vi "Pointer MAIN producer consumer.vi"() -> ()   [LabVIEW 2014]
uses:
  Ctrls/Data cluster.ctl
  <vilib>/Utility/inputDevices.llb/closeKeyboard.vi
  support/User Event - Stop/User Event - Stop.lvlib
  support/Message Queue/Message Queue.lvlib
panel:
  out "COMP-S loopback disable request":bool
  out "COMP-S ON":bool
  out "Diodes \ncable OFF":bool
  out "Version":string
  out "CloudDet\n  Active":bool
  in  "Sound":bool
  in  "Help":bool
  in  "Clouds":bool
  in  "Auto Balance":bool
  out "Loopback\n   Active":bool
  out "Clouds\n detected":bool
  in  "Loopback":bool
  out "AutoBal \n Active":bool
  in  "Tab Control":T1(tab)
  in  "Auto diode":bool
  in  "Speed Control":u8(slide)=1 min=1 max=8 step=1 scale=1.0..8.0 scale format="%1d"
  in  "PA°":u16 max=359
  in  "UP":bool caption="Solar disk to UP\n side of the image"
  in  "RIGHT":bool caption="Solar disk to RIGHT\n side of the image"
  in  "DOWN":bool caption="Solar disk to DOWN\n side of the image"
  in  "LEFT":bool caption="Solar disk to LEFT\nside of the image"
  in  "CD_sensitivity %":i8(slide)=90 min=0 max=100 scale=0.1..100.0
  out "A+    Right diode":dbl format="%#.4g"
  out "D+    Bottom diode":dbl format="%#.4g"
  out "A-    Left diode":dbl format="%#.4g"
  out "D-     Upper diode":dbl caption="D-     Upper diode \nSouth@solar disk image" format="%#.4g"
  in  "Pointer \nTolerance":i8(slide)=1 min=1 max=100 step=1 scale=1.0..11.0
  in  "Diodes ON/OFF":bool=TRUE
  out "[V]":dbl=0.0023
  out "['']":i16
  in  "Default TDMS path":string="c:\\Pointer_logs_raw\\"
  in  "VISA port":refnum<visa-resource-name>="COM4"
  in  "PA Corr°":dbl caption="PA Correction°" min=-26.3 max=26.3 step=0.1 format="%#_3g"
  out "A+":bool
  out "A-":bool caption="A+"
  out "D+":bool caption="A+"
  out "D-":bool caption="A+"
  in  "Data Logging\n     ON/OFF":bool
  in  "Loops":u8=3 min=1
  out "TDMS file name/location":path
  out "Difference Chart":T2(graph)
  out "ADC Chart":cluster{dbl, dbl, dbl, dbl}(graph)
  out "Motor Chart":cluster{dbl, i16}(graph)
  out "Output picture":picture
  in  "Active num of impls":u8
  in  "Total num of impls":u8
  out "Impulses":bool
  out "Iteractions":i32
  out "HEX Out Cmd":string=" "
  out "PA rounded":dbl
  out "Speed level":u8
  in  "A+ ADC3":dbl=0.4 step=0.0025
  in  "D+ ADC2":dbl=0.4 step=0.0025
  in  "A-  ADC1":dbl=0.4 step=0.0025
  in  "D- ADC0":dbl=0.4 step=0.0025
  in  "Diodes - Manual":bool
  out "Vertical sum":dbl
  out "Horizontal sum":dbl
  in  "ADA  level 3 [V] in":dbl=0.2 format="%#_13g"
  in  "ADA  level 2 [V] in":dbl=0.05 format="%#_13g"
  out "ADA  level 1 [V]":dbl
  out "ADA  level 2 [V]":dbl
  in  "Reverse moving":bool=TRUE caption="Reverse \nmoving"
  out "ADA  level 3 [V]":dbl
  in  "ADA  level 1 [V] in":dbl=0.0023 format="%#_13g"
  out "max time":u32 caption="max process loop time [ms]"
  in  "Total stop":bool
  # "South@solar disk image"
  # "MOVING"
  # "East@solar disk image"
  # "West@solar disk image"
  # "North@solar disk image"
  # "View from the objective lens towards the primary solar image"
  # "MEASURED  VOLTAGES"
  # "MOTOR MOVING"
  # "SETTINGS"
  # "[%]"
  # "[~]"
  # "TDMS"
  # "For testing only"
  # "RM=False\nA0 -> STOP\nA1 -> DOWN\nA2 -> UP\nA4 -> RIGHT\nA8 -> LEFT\nA5 -> DOWN/RIGHT\nA6 -> UP/RIGHT\nA9 -> DOWN/LEFT\nAA -> UP/LEFT"
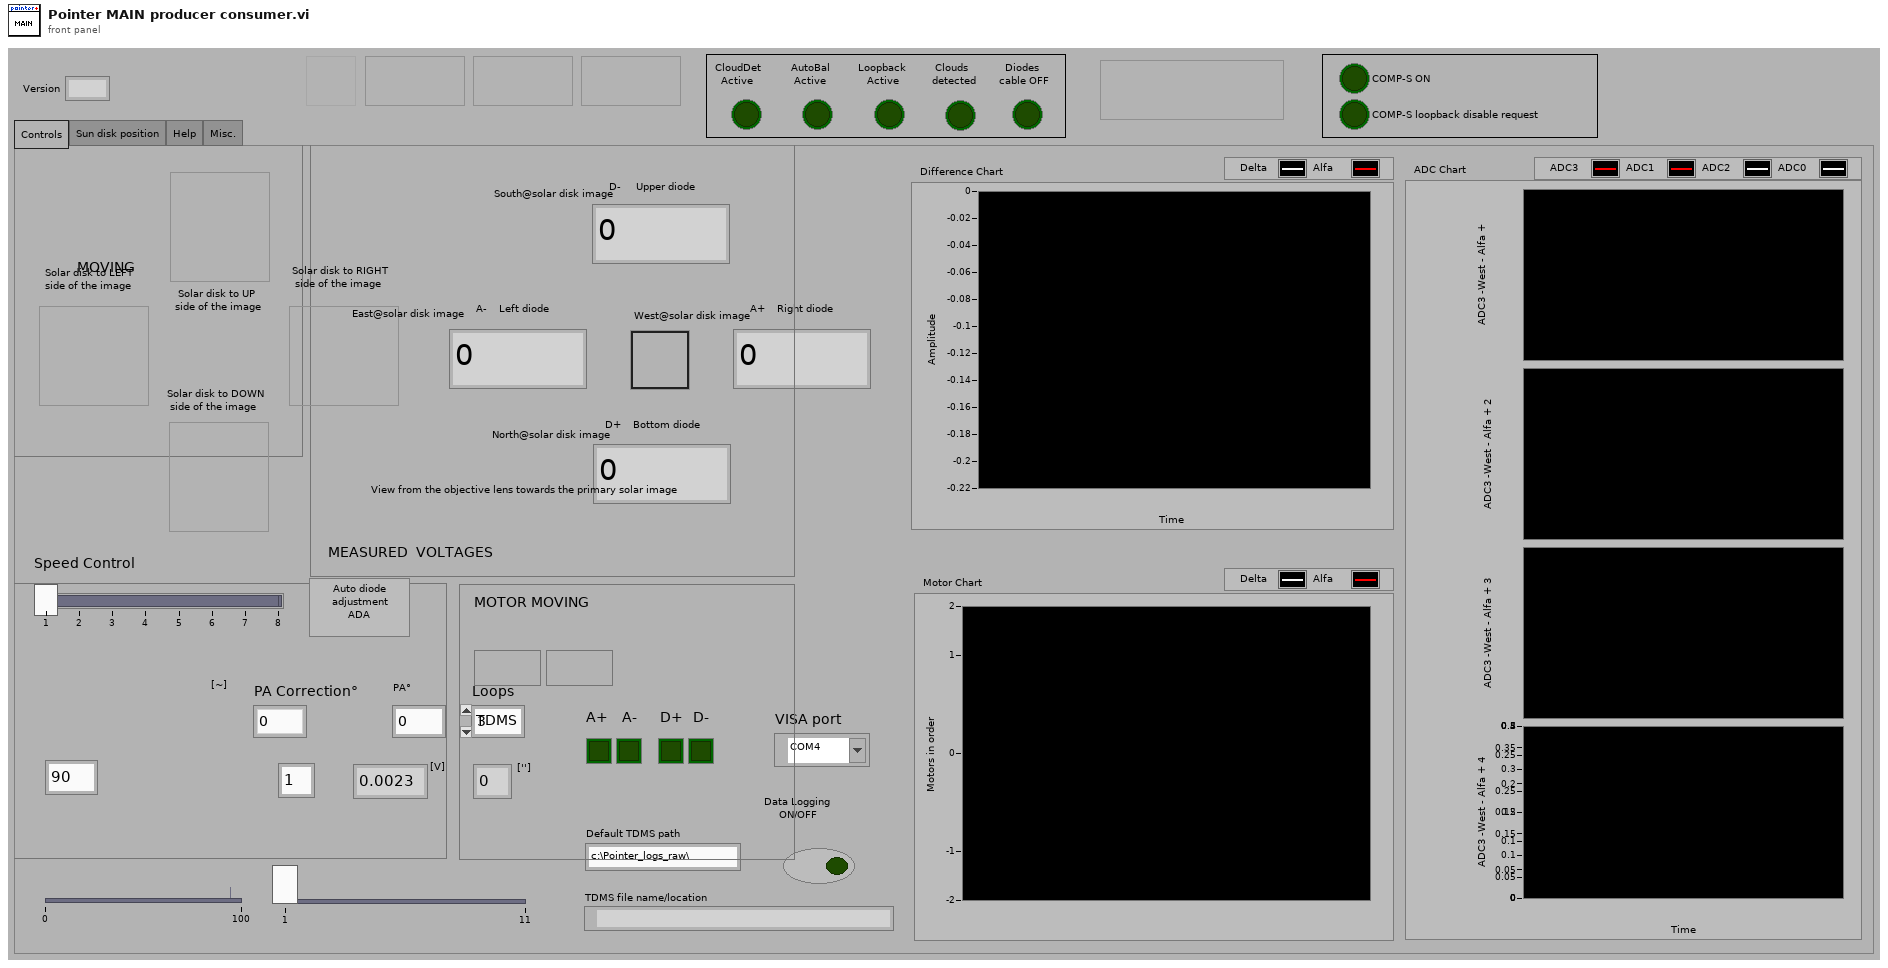
[diagram p1: front panel]
types:
  T1 = enum32{"Controls", "Sun disk position", "Help", "Misc."}
  T2 = cluster{"Vertical summary":dbl, "Horizontal summary":dbl}
  T3 = cluster{"Auto diode":refnum<vi>, "RIGHT":refnum<vi>, "UP":refnum<vi>, "LEFT":refnum<vi>, "DOWN":refnum<vi>, "Loopback":refnum<vi>, "Speed Control":refnum<vi>, "Data Log ON/OFF":refnum<vi>}
  T4 = typedef "Data cluster.ctl" = cluster{"[V]":dbl, "Vertical sum":dbl, "Horizontal sum":dbl, "auto Loopback":bool, "Auto Balance":bool, "Out Cmd":i32, "Motor Cmd":i32, "ADC Values":dbl[], "Clouds ctrl":bool, "Cloud Det":bool, "Cloud Sens":i8, "Loops":u8, "VISA res":refnum<visa-resource-name>}
  T5 = cluster{"Horizontal summary":dbl, "Vertical summary":dbl}[]
  T6 = cluster{"New ADC3":dbl, "New ADC2":dbl, dbl, dbl}[]
  T7 = typedef "LVDateTimeRec.ctl" = cluster{"fractional second":dbl, "second":i32, "minute":i32, "hour":i32, "day of month":i32, "month":i32, "year":i32, "day of week":i32, "day of year":i32, "DST":i32}
  T8 = typedef "Message Queue.lvlib/All Message Queues.ctl" = cluster{"UI":refnum<queue>}
  T9 = enum16{"0", "1", "2", "3", "4", "5", "6", "7", "8", "9", "A", "B", "C", "D", "E", "F", "G", "H", "I", "J", "K", "L", "M", "N", "O", "P", "Q", "R", "S", "T", "U", "V", "W", "X", "Y", "Z", "F1", "F2", "F3", "F4", "F5", "F6", "F7", "F8", "F9", "F10", "F11", "F12", "F13", "F14", "F15", "ADD", "BACK", "BACKSLASH", "CAPITAL", "COMMA", "DECIMAL", "DELETE", "DIVIDE", "DOWN", "END", "EQUALS", "ESCAPE", "GRAVE (`)", "HOME", "INSERT", "LBRACKET", "LCONTROL", "LEFT", "L ALT", "LSHIFT", "LWIN", "MINUS", "MULTIPLY", "NEXT", "NUMLOCK", "NUMPAD_0", "NUMPAD_1", "NUMPAD_2", "NUMPAD_3", "NUMPAD_4", "NUMPAD_5", "NUMPAD_6", "NUMPAD_7", "NUMPAD_8", "NUMPAD_9", "PAUSE", "PERIOD", "PRIOR (PG UP)", "RBRACKET", "RCONTROL", "RETURN", "RIGHT", "R ALT", "RSHIFT", "RWIN", "SCROLL", "SEMICOLON", "SLASH", "SPACE", "SUBTRACT", "TAB", "UP", "ENTER (num pad)", "' (quote)"}
  T10 = cluster{"Vertical sum":dbl, "Horizontal sum":dbl}
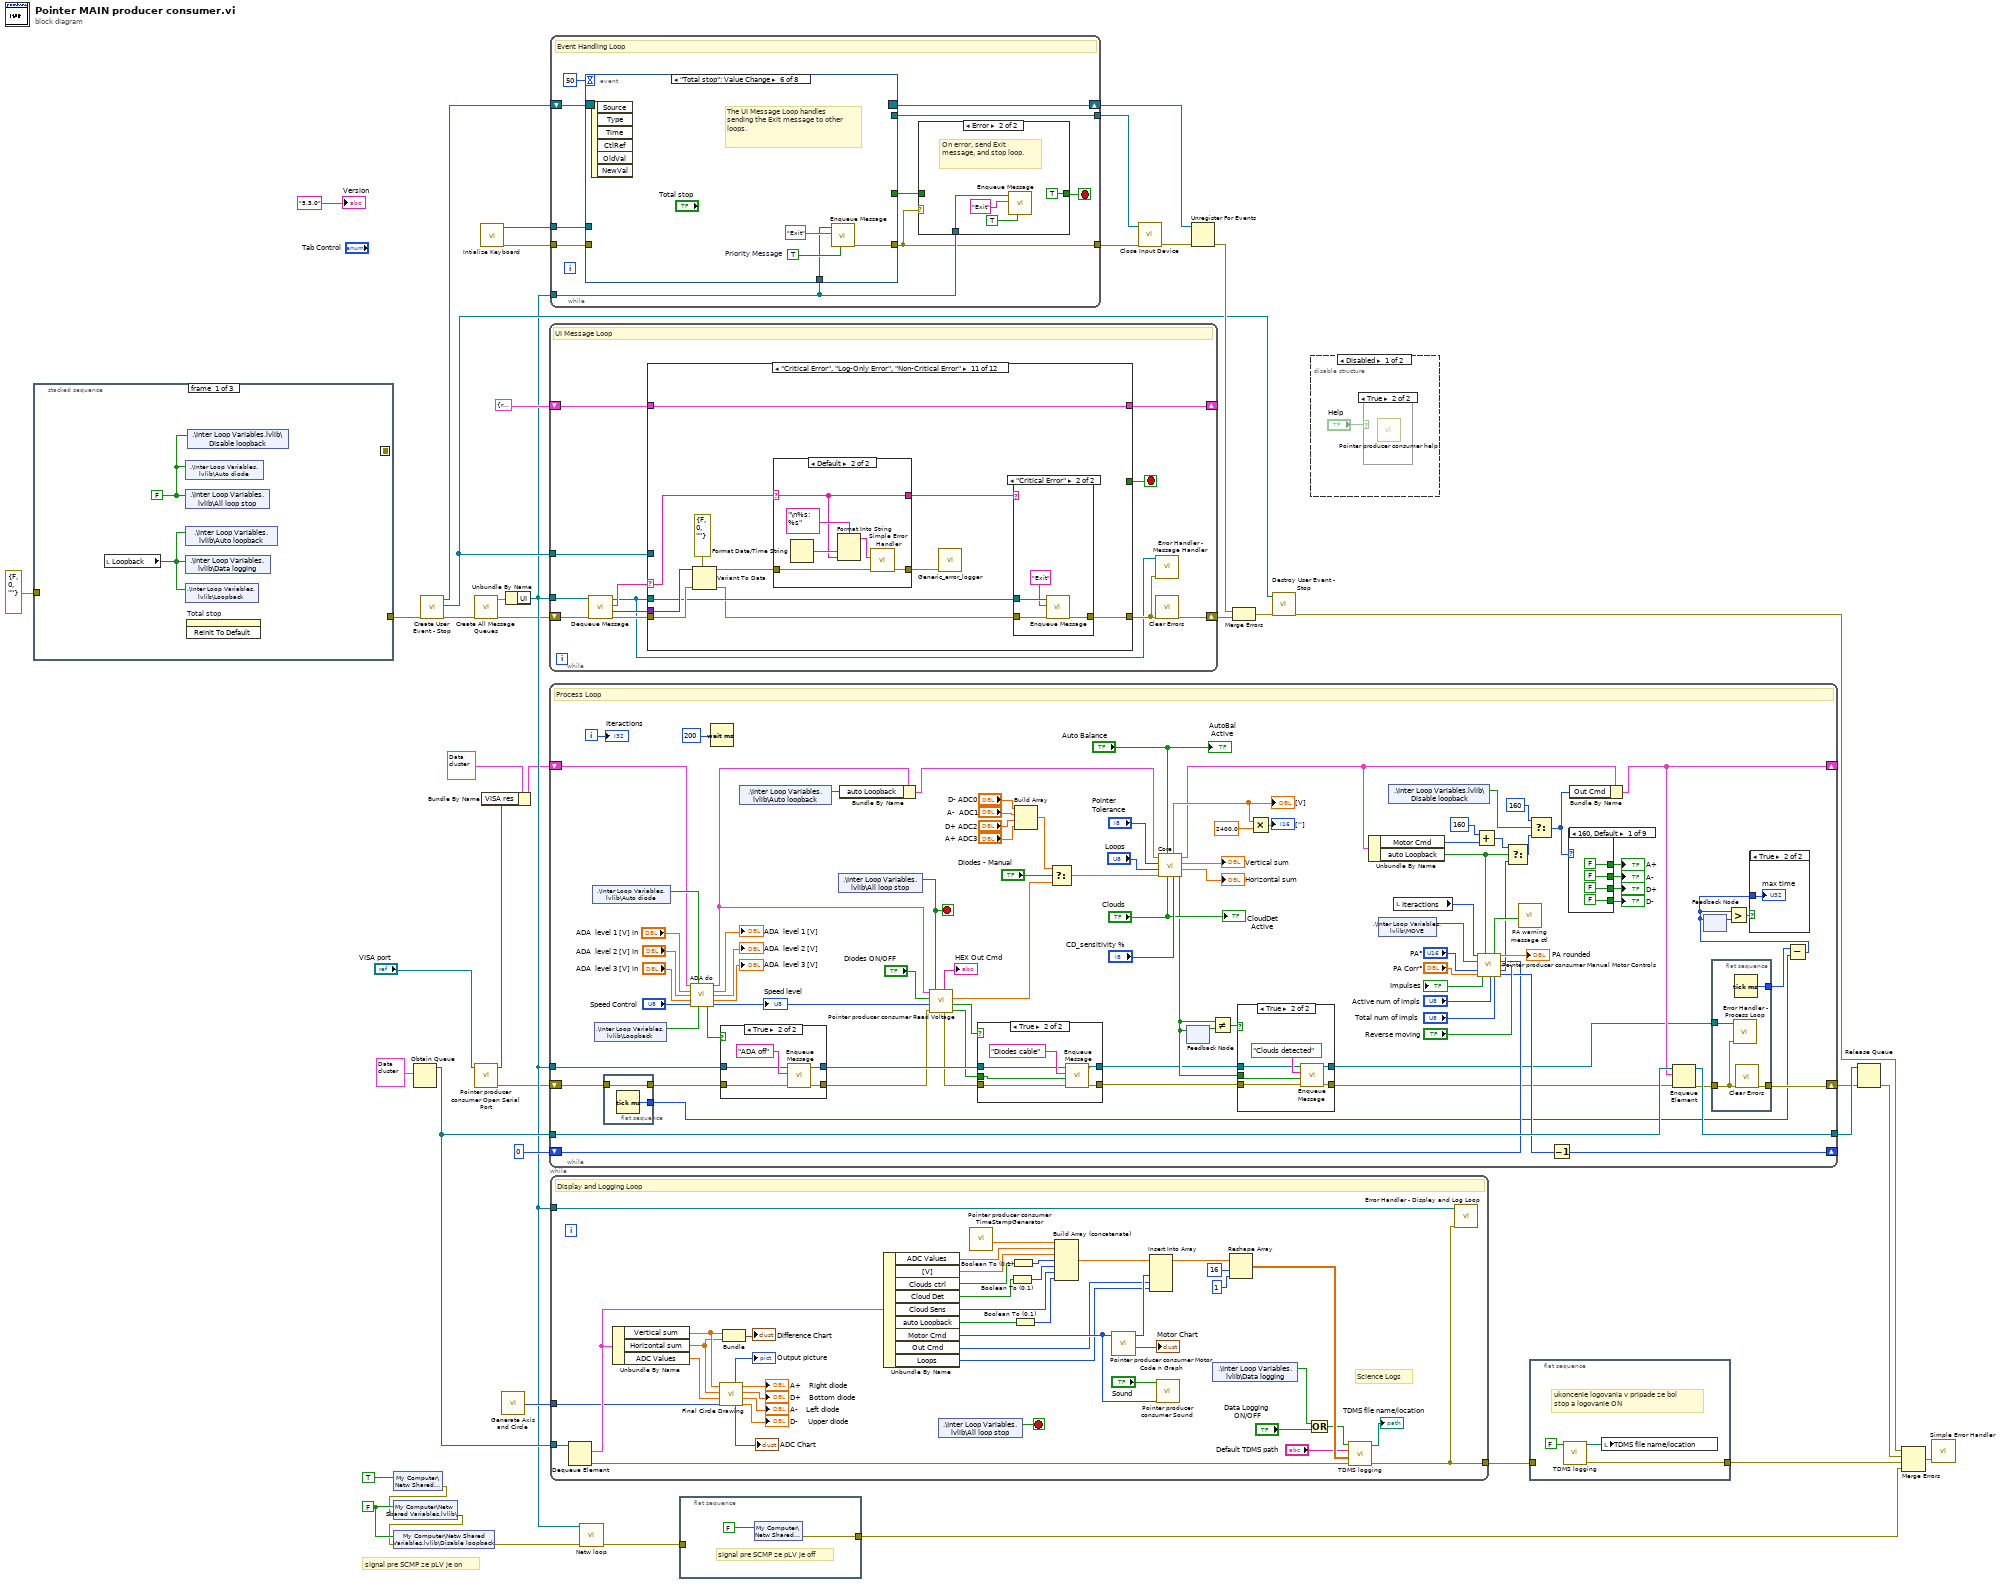
[diagram p0: block diagram]
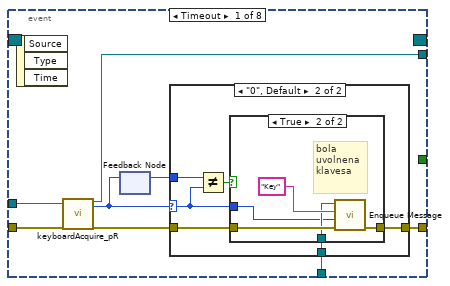
[diagram p5: hidden frame]
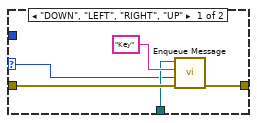
[diagram p6: hidden frame]
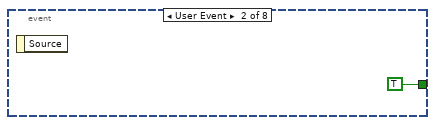
[diagram p8: hidden frame]
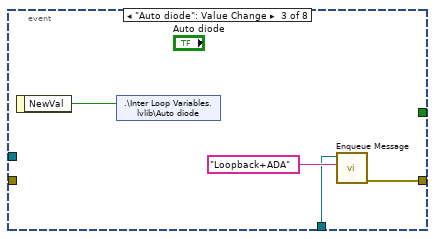
[diagram p9: hidden frame]
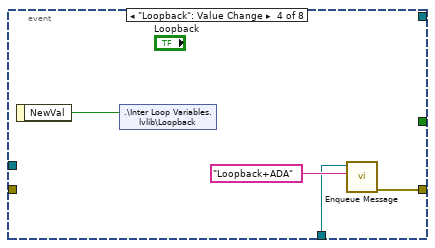
[diagram p10: hidden frame]
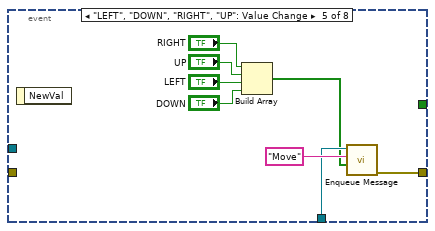
[diagram p11: hidden frame]
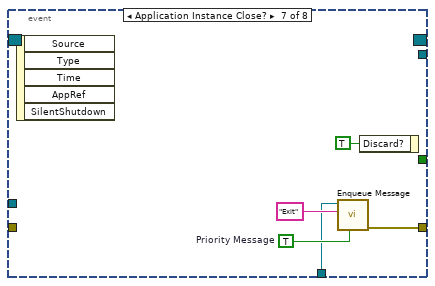
[diagram p12: hidden frame]
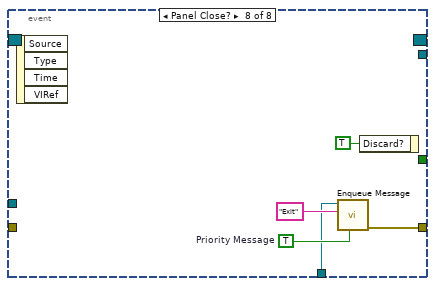
[diagram p13: hidden frame]
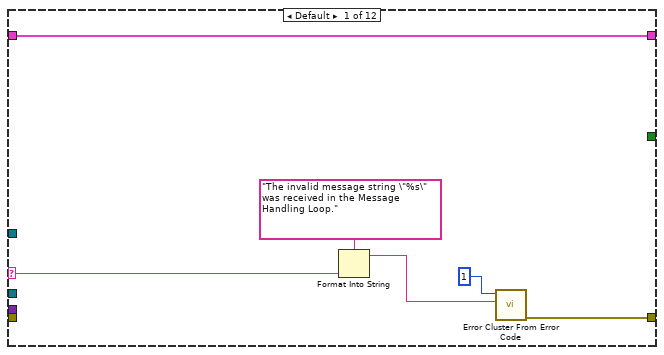
[diagram p14: hidden frame]
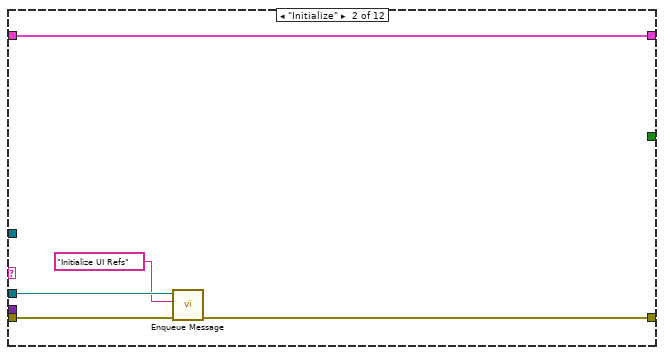
[diagram p15: hidden frame]
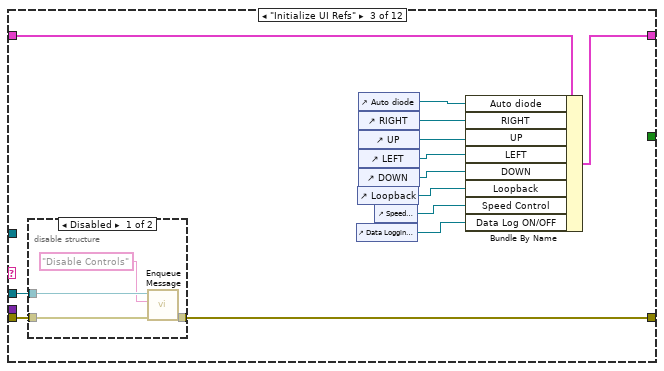
[diagram p16: hidden frame]
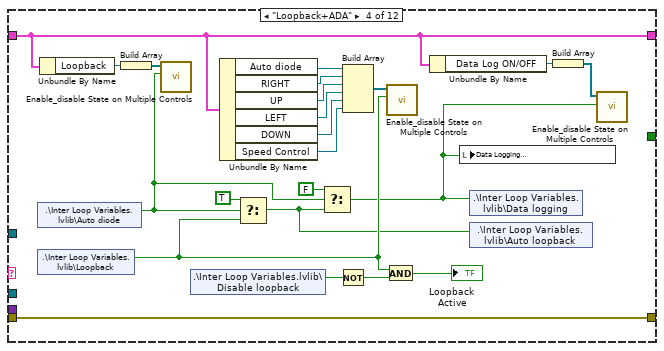
[diagram p18: hidden frame]
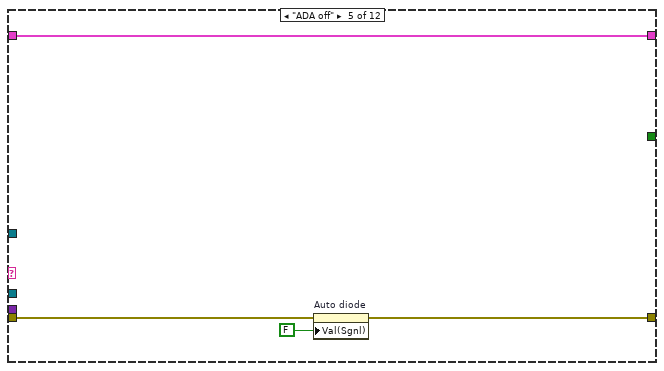
[diagram p19: hidden frame]
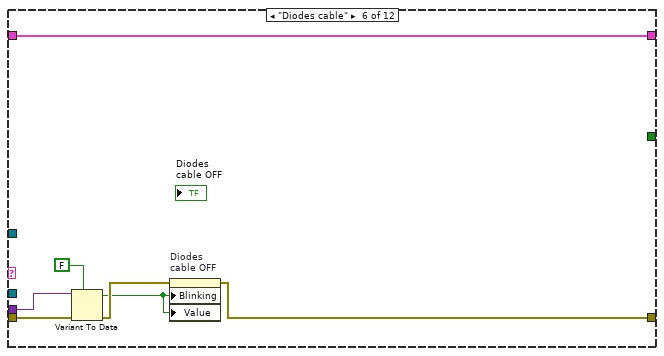
[diagram p20: hidden frame]
diagram:
  w11 = FALSE ("COMPs")
  # "signal pre SCMP ze pLV je on"
  n1 = stacked-sequence {
    seq-local: [_ w46 _] -> [_ _ w54]
    tunnel: [_ _ w57] -> w18
    tunnel: errorcluster {"status"=FALSE, "code"=0, "source"=""} ("error out") -> [_ w45 _]
    frame #0 {
      w43 = FALSE ("All loop stop")
      n2 = local read "Loopback"() -> (w44:bool)
      n3 = shared-variable ".\\Inter Loop Variables.lvlib\\Auto diode"(w43) -> ()  [unwired: 1 in, 1 out]
      n4 = shared-variable ".\\Inter Loop Variables.lvlib\\All loop stop"(w43) -> ()  [unwired: 1 in, 1 out]
      n5 = shared-variable ".\\Inter Loop Variables.lvlib\\Auto loopback"(w44) -> ()  [unwired: 1 in, 1 out]
      n6 = shared-variable ".\\Inter Loop Variables.lvlib\\Data logging"(w44) -> ()  [unwired: 1 in, 1 out]
      n7 = shared-variable ".\\Inter Loop Variables.lvlib\\Loopback"(w44) -> ()  [unwired: 1 in, 1 out]
      n8 = invoke on="Total stop" class="Bool" method="Reinit To Default"() -> ()  [unwired: 3 in, 3 out]
      n9 = shared-variable ".\\Inter Loop Variables.lvlib\\Disable loopback"(w43) -> ()  [unwired: 1 in, 1 out]
    }
    frame #1 {
      w49 = 0.200305 ("X Scale.Offset and Multiplier:Multiplier")
      # "mh v3.04: casova os -> akt cas"
      n10 = property on="Motor Chart" class="WFChart (strict)"(error in=w45, "XScale.Multiplier"=w49, "History Data"=cluster{i16, i16}[] [], "XScale.Maximum"=300.0 ("X Scale.Range:Maximum")) -> (error out=w48:errorcluster)  [unwired: 1 in, 1 out]
      n11 = property on="ADC Chart" class="WFChart (strict)"(error in=w48, "XScale.Multiplier"=w49, "History Data"=T6 []) -> (error out=w47:errorcluster)  [unwired: 1 in, 1 out]
      n12 = property on="Difference Chart" class="WFChart (strict)"(error in=w47, "XScale.Multiplier"=w49, "History Data"=T5 []) -> (error out=w46:errorcluster)  [unwired: 1 in, 1 out]
    }
    frame #2 {
      # "mh v3.04: casova os -> akt cas"
      n13 = Get Date/Time In Seconds() -> (seconds since 1Jan1904=w69:timestamp)
      n14 = Seconds To Date/Time(time stamp (now)=w69, to UTC (F)=TRUE) -> (date time rec=w68:T7)
      n15 = Unbundle(w68) -> ("second"=w62:i32, "minute"=w61:i32, "hour"=w60:i32)  [unwired: 7 out]
      n16 = Multiply(x=w60, y=60.0) -> (x*y=w67:dbl)
      n17 = Add(x=w61, y=w67) -> (x+y=w63:dbl)
      n18 = Multiply(x=w63, y=60.0) -> (x*y=w65:dbl)
      n19 = Add(x=w62, y=w65) -> (x+y=w58:dbl)
      n20 = property on="ADC Chart" class="WFChart (strict)"(error in=w54, "XScale.Offset"=w58) -> (error out=w55:errorcluster)  [unwired: 1 in, 1 out]
      n21 = property on="Difference Chart" class="WFChart (strict)"(error in=w55, "XScale.Offset"=w58) -> (error out=w56:errorcluster)  [unwired: 1 in, 1 out]
      n22 = property on="Motor Chart" class="WFChart (strict)"(error in=w56, "XScale.Offset"=w58) -> (error out=w57:errorcluster)  [unwired: 1 in, 1 out]
    }
  }
  n23 = shared-variable "My Computer\\Netw Shared Variables.lvlib\\pLV"(TRUE ("pLV")) -> (error out=w10:errorcluster)  [unwired: 1 in]
  n24 = shared-variable "My Computer\\Netw Shared Variables.lvlib\\COMPs"(w11, error in=w10) -> (error out=w9:errorcluster)
  n25 = shared-variable "My Computer\\Netw Shared Variables.lvlib\\Disable loopback"(w11, error in=w9) -> (error out=w8:errorcluster)
  n26 = Obtain Queue(element data type=T4 {"[V]"=0.0, "Vertical sum"=0.0, "Horizontal sum"=0.0, "auto Loopback"=FALSE, "Auto Balance"=FALSE, "Out Cmd"=0, "Motor Cmd"=0, "ADC Values"=[], "Clouds ctrl"=FALSE, "Cloud Det"=FALSE, "Cloud Sens"=0, "Loops"=0, "VISA res"="COM3"}) -> (queue out=w42:refnum<queue>)  [unwired: 4 in, 2 out]
  n27 = call "Create User Event - Stop.vi"("error in (no error)"=w18) -> ("error out"=w29:errorcluster, "User Event - Stop"=w24:refnum<user-event>, "Stop Event Registration Refnum"=w28:refnum<event-registration>)  [unwired: 8 in]
  n28 = call "Create All Message Queues.vi"("error in (no error)"=w29) -> ("error out"=w2:errorcluster, "Message Queues out"=w32:T8)  [unwired: 9 in]
  n29 = call "Pointer producer consumer Open Serial Port.vi"("VISA resource name"="VISA port") -> ("error out"=w1:errorcluster, "VISA resource name out"=w3:refnum<visa-resource-name>)  [unwired: 9 in]
  n30 = call <vilib>:"Intialize Keyboard.vi"() -> ("error out"=w21:errorcluster, "device ID"=w20:refnum<k1>)  [unwired: 1 in, 9 out]
  n31 = Bundle By Name(cluster=T4 {"[V]"=0.0, "Vertical sum"=0.0, "Horizontal sum"=0.0, "auto Loopback"=FALSE, "Auto Balance"=FALSE, "Out Cmd"=0, "Motor Cmd"=0, "ADC Values"=[], "Clouds ctrl"=FALSE, "Cloud Det"=FALSE, "Cloud Sens"=0, "Loops"=0, "VISA res"="COM3"}, "VISA res"=w3) -> (w4:T4)
  n32 = call "Generate Axis and Circle.vi"() -> ("Output picture"=w40:picture)  [unwired: 1 in]
  n33 = Unbundle By Name(w32) -> ("UI"=w13:refnum<queue>)
  n34 = while {
    shift-right: [w76] -> w31
    shift-left: w2 -> [w81]
    tunnel: w13 -> [w77]
    shift-right: [w72] -> _
    shift-left: T3 {"Auto diode"=refnum, "RIGHT"=refnum, "UP"=refnum, "LEFT"=refnum, "DOWN"=refnum, "Loopback"=refnum, "Speed Control"=refnum, "Data Log ON/OFF"=refnum} -> [w73]
    tunnel: w24 -> [w70]
    stop <- w71 stop-if-true
    # "UI Message Loop"
    n35 = call "Dequeue Message.vi"("error in (no error)"=w81, "Message Queue"=w77) -> ("error out"=w80:errorcluster, "Message Data"=w79:variant, "Message"=w78:string, "dup Message Queue"=w74:refnum<queue>)  [unwired: 6 in]
    n36 = case shown="\"Critical Error\", \"Log-Only Error\", \"Non-Critical Error\"" w78 {
      selector: w78 -> [w84 _ _ _ _ _ _ _ _ _ w200 _]
      tunnel: w80 -> [_ w91 w104 w130 w134 w142 w149 w158 w186 w197 w207 w230]
      tunnel: w79 -> [_ _ _ _ _ w141 w148 w157 w185 w196 w205 _]
      tunnel: w74 -> [_ w92 w105 _ _ _ _ w152 _ w188 w204 w225]
      tunnel: [w83 w90 w103 w130 w133 w137 w145 w153 w183 w189 w206 w228] -> w75
      tunnel: w73 -> [w82 w88 w94 w118 w136 w143 w150 w159 w187 w198 w209 w232]
      tunnel: [w82 w88 w93 w118 w136 w143 w150 w159 w187 w198 w209 w232] -> w72
      tunnel: [_ _ _ _ _ _ _ _ _ _ _ TRUE] -> w71
      tunnel: w70 -> [_ _ _ _ _ _ _ _ _ _ _ w227]
      frame Default {
        n37 = Format Into String(format string="The invalid message string \"%s\" was received in the Message Handling Loop." ("Invalid Message Loop Message"), w84) -> (resulting string=w85:string)  [unwired: 2 in, 1 out]
        n38 = call <vilib>:"Error Cluster From Error Code.vi"("error message (\"\")"=w85, "error code (0)"=1) -> ("error out"=w83:errorcluster)  [unwired: 7 in]
      }
      frame "Initialize" {
        n39 = call "Enqueue Message.vi"("error in (no error)"=w91, "Message"="Initialize UI Refs", "Message Queue"=w92) -> ("error out"=w90:errorcluster)  [unwired: 7 in, 1 out]
      }
      frame "Initialize UI Refs" {
        n40 = disable-structure shown="Disabled" {
          disable-tunnel: w105 -> [w109 _]
          disable-tunnel: w104 -> [w108 w110]
          disable-tunnel: [w107 w110] -> w103
          frame Disabled {
            n41 = call "Enqueue Message.vi"("error in (no error)"=w108, "Message"="Disable Controls", "Message Queue"=w109) -> ("error out"=w107:errorcluster)  [unwired: 7 in, 1 out]
          }
          frame Enabled {
          }
        }
        n42 = control-ref of="Data Logging ON/OFF"() -> (w102:refnum<vi>)
        n43 = control-ref of="Loopback"() -> (w100:refnum<vi>)
        n44 = control-ref of="Auto diode"() -> (w95:refnum<vi>)
        n45 = control-ref of="RIGHT"() -> (w96:refnum<vi>)
        n46 = control-ref of="UP"() -> (w97:refnum<vi>)
        n47 = control-ref of="LEFT"() -> (w98:refnum<vi>)
        n48 = control-ref of="DOWN"() -> (w99:refnum<vi>)
        n49 = control-ref of="Speed Control"() -> (w101:refnum<vi>)
        n50 = Bundle By Name(cluster=w94, "Auto diode"=w95, "RIGHT"=w96, "UP"=w97, "LEFT"=w98, "DOWN"=w99, "Loopback"=w100, "Speed Control"=w101, "Data Log ON/OFF"=w102) -> (w93:T3)
      }
      frame "Loopback+ADA" {
        n51 = shared-variable ".\\Inter Loop Variables.lvlib\\Auto diode"() -> (w127:bool)  [unwired: 1 in, 1 out]
        n52 = shared-variable ".\\Inter Loop Variables.lvlib\\Loopback"() -> (w119:bool)  [unwired: 1 in, 1 out]
        n53 = Unbundle By Name(w118) -> ("Loopback"=w132:refnum<vi>)
        n54 = Build Array(w132) -> (w131:refnum<vi>[])
        n55 = call "Enable_disable State on Multiple Controls.vi"("Disable control?"=w127, "Controls"=w131) -> ()  [unwired: 9 in, 1 out]
        n56 = shared-variable ".\\Inter Loop Variables.lvlib\\Disable loopback"() -> (w112:bool)  [unwired: 1 in, 1 out]
        n57 = Unbundle By Name(w118) -> ("Auto diode"=w121:refnum<vi>, "RIGHT"=w122:refnum<vi>, "UP"=w123:refnum<vi>, "LEFT"=w124:refnum<vi>, "DOWN"=w125:refnum<vi>, "Speed Control"=w126:refnum<vi>)
        n58 = Select(t=TRUE, s=w127, f=w119) -> (s? t:f=w115:bool)
        n59 = Select(t=FALSE, s=w127, f=w115) -> (s? t:f=w114:bool)
        n60 = Not(x=w112) -> (.not. x?=w111:bool)
        n61 = Build Array(w121, w122, w123, w124, w125, w126) -> (w120:refnum<vi>[])
        n62 = And(x=w119, y=w111) -> (x .and. y?=→"Loopback\n   Active":bool)
        n63 = call "Enable_disable State on Multiple Controls.vi"("Disable control?"=w119, "Controls"=w120) -> ()  [unwired: 9 in, 1 out]
        n64 = Unbundle By Name(w118) -> ("Data Log ON/OFF"=w116:refnum<vi>)
        n65 = local write "Data Logging\n     ON/OFF"(w114) -> ()
        n66 = shared-variable ".\\Inter Loop Variables.lvlib\\Data logging"(w114) -> ()  [unwired: 1 in, 1 out]
        n67 = shared-variable ".\\Inter Loop Variables.lvlib\\Auto loopback"(w115) -> ()  [unwired: 1 in, 1 out]
        n68 = Build Array(w116) -> (w117:refnum<vi>[])
        n69 = call "Enable_disable State on Multiple Controls.vi"("Disable control?"=w114, "Controls"=w117) -> ()  [unwired: 9 in, 1 out]
      }
      frame "ADA off" {
        n70 = property on="Auto diode" class="Bool (strict)"(error in=w134, "Val(Sgnl)"=FALSE) -> (error out=w133:errorcluster)  [unwired: 1 in, 1 out]
      }
      frame "Diodes cable" {
        n71 = Variant To Data(error in=w142, type=FALSE ("Diodes \ncable OFF"), Variant=w141) -> (data=w138:bool, error out=w139:errorcluster)
        n72 = property on="Diodes \ncable OFF" class="Bool (strict)"(error in=w139, "Blinking"=w138, "Value"=w138) -> (error out=w137:errorcluster)  [unwired: 1 in, 1 out]
      }
      frame "Clouds detected" {
        n73 = Variant To Data(error in=w149, type=FALSE ("Diodes \ncable OFF"), Variant=w148) -> (data=w144:bool, error out=w146:errorcluster)
        n74 = property on="Clouds\n detected" class="Bool (strict)"(error in=w146, "Blinking"=w144, "Value"=w144) -> (error out=w145:errorcluster)  [unwired: 1 in, 1 out]
      }
      frame "Key" {
        n75 = shared-variable ".\\Inter Loop Variables.lvlib\\Auto loopback"() -> (w151:bool)  [unwired: 1 in, 1 out]
        n76 = Variant To Data(error in=w158, type=T9."0" ("key pressed"), Variant=w157) -> (data=w155:T9, error out=w154:errorcluster)
        n77 = case shown="False" w151 {
          tunnel: w155 -> [w169 _]
          tunnel: w154 -> [w163 w181]
          tunnel: [w162 w181] -> w153
          tunnel: w152 -> [w161 _]
          frame False {
            n78 = case shown="\"0\", Default" w169 {
              tunnel: [w172 w174 w176 w178 w179] -> w165
              tunnel: [w172 w174 w176 w177 w180] -> w166
              tunnel: [w172 w173 w176 w178 w180] -> w168
              tunnel: [w172 w174 w175 w178 w180] -> w167
              tunnel: TRUE ("Solar disk to LEFT\nside of the image") -> [_ w173 w175 w177 w179]
              tunnel: FALSE ("Solar disk to LEFT\nside of the image") -> [w172 w174 w176 w178 w180]
              frame "0", Default {
                # "bola uvolnena klavesa"
              }
              frame "RIGHT" {
              }
              frame "UP" {
              }
              frame "LEFT" {
              }
              frame "DOWN" {
              }
            }
            n79 = local write "RIGHT"(w168) -> ()
            n80 = local write "UP"(w167) -> ()
            n81 = local write "LEFT"(w166) -> ()
            n82 = local write "DOWN"(w165) -> ()
            n83 = Build Array(w168, w167, w166, w165) -> (w160:bool[])
            n84 = call "Enqueue Message.vi"("error in (no error)"=w163, "Message Data"=w160, "Message"="Move", "Message Queue"=w161) -> ("error out"=w162:errorcluster)  [unwired: 6 in, 1 out]
          }
          frame True {
          }
        }
      }
      frame "Move" {
        n85 = Variant To Data(error in=w186, type=bool[] [TRUE, TRUE, TRUE, TRUE], Variant=w185) -> (data=w182:bool[], error out=w183:errorcluster)
        n86 = shared-variable ".\\Inter Loop Variables.lvlib\\MOVE"(w182) -> ()  [unwired: 1 in, 1 out]
      }
      frame "Netw Loopback" {
        # "volanie len kvoli update\n indikatoru loopback"
        n87 = Variant To Data(error in=w197, type=bool[] [TRUE, TRUE], Variant=w196) -> (data=w194:bool[], error out=w190:errorcluster)
        n88 = Index Array(array=w194) -> (element #1=→"COMP-S ON":bool, element #2=→"COMP-S loopback disable request":bool)  [unwired: 2 in]
        n89 = call "Enqueue Message.vi"("error in (no error)"=w190, "Message"="Loopback+ADA", "Message Queue"=w188) -> ("error out"=w189:errorcluster)  [unwired: 7 in, 1 out]
      }
      frame "Critical Error", "Log-Only Error", "Non-Critical Error" {
        n90 = Variant To Data(error in=w207, type=errorcluster {"status"=FALSE, "code"=0, "source"=""} ("error constant"), Variant=w205) -> (data=w202:errorcluster, error out=w203:errorcluster)
        n91 = case shown="Default" w200 {
          selector: w200 -> [w210 w212]
          tunnel: w202 -> [w211 w214]
          tunnel: [w211 w213] -> w201
          tunnel: [w210 w212] -> w199
          frame "Log-Only Error" {
          }
          frame Default {
            n92 = Format Date/Time String() -> (date/time string=w216:string)  [unwired: 3 in]
            n93 = Format Into String(format string="\n%s: %s", w216, w212) -> (resulting string=w215:string)  [unwired: 2 in, 1 out]
            n94 = call <vilib>:"Simple Error Handler.vi"("error source (\" \")"=w215, "error in (no error)"=w214) -> ("error out"=w213:errorcluster)  [unwired: 3 in, 4 out]
          }
        }
        n95 = call "Generic_error_logger.vi"("Error to log"=w201) -> ()  [unwired: 10 in, 1 out]
        n96 = case shown="\"Critical Error\"" w199 {
          tunnel: w203 -> [w218 w222]
          tunnel: w204 -> [_ w220]
          tunnel: [w218 w221] -> w206
          frame Default {
          }
          frame "Critical Error" {
            n97 = call "Enqueue Message.vi"("error in (no error)"=w222, "Message"="Exit", "Message Queue"=w220) -> ("error out"=w221:errorcluster)  [unwired: 7 in, 1 out]
          }
        }
      }
      frame "Exit" {
        w223 = FALSE ("COMP-S connected")
        # "Stop Event Handling Loop"
        # "Release the UI Message queue reference"
        # "Stop UI Message Loop"
        n98 = call "Fire User Event - Stop.vi"("User Event - Stop"=w227) -> ("error out"=w226:errorcluster)  [unwired: 10 in]
        n99 = Release Queue(queue=w225, error in (no error)=w230) -> (error out=w231:errorcluster)  [unwired: 1 in, 2 out]
        n100 = shared-variable ".\\Inter Loop Variables.lvlib\\All loop stop"(TRUE ("All loop stop")) -> ()  [unwired: 1 in, 1 out]
        n101 = local write "COMP-S loopback disable request"(w223) -> ()
        n102 = local write "COMP-S ON"(w223) -> ()
        n103 = Merge Errors(w226, w231) -> (w228:errorcluster)
      }
    }
    n104 = call "Error Handler - Message Handler.vi"("error in (no error)"=w75, "Message Queue"=w74) -> ()  [unwired: 9 in, 1 out]
    n105 = call <vilib>:"Clear Errors.vi"("error in (no error)"=w75) -> ("error out"=w76:errorcluster)  [unwired: 5 in, 1 out]
  }
  n106 = while {
    tunnel: w42 -> [w322]
    tunnel: [w321] -> w41
    shift-right: [w287] -> _
    shift-left: w4 -> [w246]
    shift-right: [w282] -> w37
    shift-left: w1 -> [w277]
    shift-right: [w290] -> _
    shift-left: 0 -> [w289]
    tunnel: w13 -> [w257]
    i -> [w320]
    stop <- w238 stop-if-true
    # "Process Loop"
    n107 = shared-variable ".\\Inter Loop Variables.lvlib\\Auto diode"() -> (w247:bool)  [unwired: 1 in, 1 out]
    n108 = shared-variable ".\\Inter Loop Variables.lvlib\\Loopback"() -> (w264:bool)  [unwired: 1 in, 1 out]
    n109 = flat-sequence {
      tunnel: [w332] -> w251
      tunnel: w277 -> [w332]
      tunnel: [w331] -> w250
      frame #0 {
        n110 = Tick Count (ms)() -> (millisecond timer value=w331:u32)
      }
    }
    n111 = call "ADA do.vi"("Data in"=w246, "Auto diode"=w247, "ADA  level 1 [V] in"="ADA  level 1 [V] in", "ADA  level 2 [V] in"="ADA  level 2 [V] in", "ADA  level 3 [V] in"="ADA  level 3 [V] in", "Speed Control in"="Speed Control", "Loopback"=w264) -> ("ADA off request"=w310:bool, "Data out"=w235:T4, "ADA  level 1 [V]"=→"ADA  level 1 [V]":dbl, "ADA  level 2 [V]"=→"ADA  level 2 [V]":dbl, "ADA  level 3 [V]"=→"ADA  level 3 [V]":dbl, "Speed Control out"=w233:u8)  [unwired: 3 in]
    "Speed level" <- w233
    n112 = Wait (ms)(milliseconds to wait=u32 200 ("Wait")) -> ()  [unwired: 1 out]
    n113 = case shown="True" w310 {
      tunnel: w257 -> [w383 w387]
      tunnel: [w383 w386] -> w256
      tunnel: [w382 w385] -> w237
      tunnel: w251 -> [w382 w384]
      frame False {
      }
      frame True {
        n114 = call "Enqueue Message.vi"("error in (no error)"=w384, "Message"="ADA off", "Message Queue"=w387) -> ("error out"=w385:errorcluster, "dup Message Queue"=w386:refnum<queue>)  [unwired: 7 in]
      }
    }
    n115 = shared-variable ".\\Inter Loop Variables.lvlib\\Auto loopback"() -> (w265:bool)  [unwired: 1 in, 1 out]
    n116 = shared-variable ".\\Inter Loop Variables.lvlib\\All loop stop"() -> (w238:bool)  [unwired: 1 in, 1 out]
    n117 = Bundle By Name(cluster=w235, "auto Loopback"=w265) -> (w245:T4)
    n118 = call "Pointer producer consumer Read Voltage.vi"("Total Stop"=w238, "error in (no error)"=w237, "Speed"=w233, "Diodes ON/OFF"="Diodes ON/OFF", "Data in"=w235) -> ("Diods cable OFF status"=w254:bool, "Diods cable OFF status request"=w255:bool, "ADC votlages"=w312:dbl[], "error out"=w236:errorcluster, "Motor Cmd"=→"HEX Out Cmd":string)  [unwired: 2 in]
    n119 = case shown="True" w255 {
      tunnel: w256 -> [w324 w329]
      tunnel: w236 -> [w323 w328]
      tunnel: w254 -> [_ w327]
      tunnel: [w324 w326] -> w253
      tunnel: [w323 w325] -> w252
      frame False {
      }
      frame True {
        n120 = call "Enqueue Message.vi"("error in (no error)"=w328, "Message Data"=w327, "Message"="Diodes cable", "Message Queue"=w329) -> ("error out"=w325:errorcluster, "dup Message Queue"=w326:refnum<queue>)  [unwired: 6 in]
      }
    }
    n121 = Build Array("D- ADC0", "A-  ADC1", "D+ ADC2", "A+ ADC3") -> (w314:dbl[])
    n122 = Select(t=w314, s="Diodes - Manual", f=w312) -> (s? t:f=w276:dbl[])
    n123 = call "Core.vi"("CD_sensitivity %"="CD_sensitivity %", "Clouds"="Clouds", "Auto Balance"="Auto Balance", "Real-time Values"=w276, "Loops"="Loops", "Pointer Tolerance"="Pointer \nTolerance", "Data in"=w245) -> ("Clouds detected"=w270:bool, "Horizontal sum"=→"Horizontal sum":dbl, "Vertical sum"=→"Vertical sum":dbl, "Data out"=w266:T4, "[V]"=w273:dbl)
    "[V]" <- w273
    n124 = feedback #1() -> (w285:bool)  [unwired: 1 in]
    n125 = feedback-in #1(w270) -> ()
    n126 = Not Equal?(x=w270, y=w285) -> (x != y?=w284:bool)
    n127 = case shown="True" w284 {
      tunnel: [w339 w341] -> w249
      tunnel: w270 -> [_ w342]
      tunnel: w253 -> [w338 w344]
      tunnel: w252 -> [w339 w343]
      tunnel: [w338 w340] -> w244
      frame False {
      }
      frame True {
        n128 = call "Enqueue Message.vi"("error in (no error)"=w343, "Message Data"=w342, "Message"="Clouds detected", "Message Queue"=w344) -> ("error out"=w341:errorcluster, "dup Message Queue"=w340:refnum<queue>)  [unwired: 6 in]
      }
    }
    n129 = Multiply(x=w273, y=2400.0) -> (x*y=→"['']":dbl)
    n130 = Unbundle By Name(w266) -> ("Motor Cmd"=w294:i32, "auto Loopback"=w288:bool)
    n131 = shared-variable ".\\Inter Loop Variables.lvlib\\MOVE"() -> (w248:bool[])  [unwired: 1 in, 1 out]
    n132 = shared-variable ".\\Inter Loop Variables.lvlib\\Disable loopback"() -> (w240:bool)  [unwired: 1 in, 1 out]
    n133 = local read "Iteractions"() -> (w301:i32)
    n134 = Add(x=160 ("y"), y=w294) -> (x+y=w299:i32)
    n135 = call "Pointer producer consumer Manual Motor Controls.vi"("Iteraction Counter"=w301, "loopback"=w288, "Input Array"=w248, "Impulse IN"=w289, "Reverse moving"="Reverse moving", "PA°"="PA°", "PA Correction°"="PA Corr°", "No. Impulses"="Active num of impls", "Modulo num"="Total num of impls") -> ("get info?"=w300:bool, "PA rounded"=→"PA rounded":dbl, "Output Number"=w292:i32, "Impulses"=→"Impulses":bool, "Impulse OUT"=w291:i32)  [unwired: 2 in]
    n136 = Select(t=w299, s=w288, f=w292) -> (s? t:f=w243:i32)
    n137 = call "PA warning message ctl.vi"("get info?"=w300) -> ()  [unwired: 11 in]
    n138 = Select(t=160 ("y"), s=w240, f=w243) -> (s? t:f=w242:i32)
    n139 = Decrement(x=w291) -> (x-1=w290:i32)
    n140 = case shown="160, Default" w242 {
      tunnel: [FALSE FALSE FALSE TRUE FALSE TRUE TRUE FALSE FALSE] -> w298
      tunnel: [FALSE FALSE FALSE FALSE TRUE FALSE FALSE TRUE TRUE] -> w297
      tunnel: [FALSE FALSE TRUE FALSE FALSE FALSE TRUE FALSE TRUE] -> w296
      tunnel: [FALSE TRUE FALSE FALSE FALSE TRUE FALSE TRUE FALSE] -> w295
      frame 160, Default {
      }
      frame 161 {
      }
      frame 162 {
      }
      frame 164 {
      }
      frame 168 {
      }
      frame 165 {
      }
      frame 166 {
      }
      frame 169 {
      }
      frame 170 {
      }
    }
    "A+" <- w298
    "A-" <- w297
    "D+" <- w296
    "D-" <- w295
    n141 = Bundle By Name(cluster=w266, "Out Cmd"=w242) -> (w287:T4)
    n142 = Enqueue Element(queue=w322, element=w287, error in (no error)=w249) -> (queue out=w321:refnum<queue>, error out=w283:errorcluster)  [unwired: 1 in, 1 out]
    n143 = feedback #2() -> (w280:u32)  [unwired: 1 in]
    n144 = flat-sequence {
      tunnel: [w336] -> w282
      tunnel: w283 -> [w335]
      tunnel: [w337] -> w281
      tunnel: w244 -> [w334]
      frame #0 {
        n145 = call "Error Handler - Process Loop.vi"("error in (no error)"=w335, "Message Queue"=w334) -> ()  [unwired: 9 in, 1 out]
        n146 = Tick Count (ms)() -> (millisecond timer value=w337:u32)
        n147 = call <vilib>:"Clear Errors.vi"("error in (no error)"=w335) -> ("error out"=w336:errorcluster)  [unwired: 5 in, 1 out]
      }
    }
    n148 = Subtract(x=w281, y=w250) -> (x-y=w279:u32)
    n149 = feedback-in #2(w279) -> ()
    n150 = Greater?(x=w279, y=w280) -> (0:w278:bool)
    n151 = case shown="True" w278 {
      tunnel: w279 -> [_ w333]
      frame False {
      }
      frame True {
        "max time" <- w333
      }
    }
    "Iteractions" <- w320
    "AutoBal \n Active" <- "Auto Balance"
    "CloudDet\n  Active" <- "Clouds"
  }
  n152 = while {
    shift-right: [w397] -> w27
    shift-left: w28 -> [w398]
    tunnel: w13 -> [w393]
    tunnel: w20 -> [w391]
    tunnel: [w390] -> w19
    tunnel: w21 -> [w392]
    tunnel: [w389] -> w17
    stop <- w396 stop-if-true
    # "Event Handling Loop"
    n153 = event shown="[5] \"Total stop\": Value Change" {
      selector: w398 -> [_ _ _ _ _ _ _ _]
      dyn-events: [_ _ _ _ _ _ _ _] -> w397
      timeout: 50 -> [_ _ _ _ _ _ _ _]
      tunnel: [_ TRUE ("Discard?") _ _ _ _ _ _] -> w395
      tunnel: [w408 _ w432 w436 w444 w447 w452 w457] -> w389
      tunnel: w393 -> [w406 _ w430 w434 w443 w446 w451 w456]
      tunnel: w392 -> [w411 _ _ _ _ _ _ _]
      tunnel: w391 -> [w410 _ _ _ _ _ _ _]
      tunnel: [w409 _ _ _ _ _ _ _] -> w390
      event Timeout {
        n154 = event-data() -> ()  [unwired: 1 in, 3 out]
        n155 = call "keyboardAcquire_pR.vi"("device ID"=w410, "error in (no error)"=w411) -> ("device ID"=w409:refnum<k1>, "key pressed"=w404:T9, "error out"=w407:errorcluster)  [unwired: 15 in]
        n156 = feedback-in #3(w404) -> ()
        n157 = feedback #3() -> (w405:T9)  [unwired: 1 in]
        n158 = case shown="\"0\", Default" w404 {
          selector: w404 -> [w412 w417]
          tunnel: [w415 w422] -> w408
          tunnel: w407 -> [w414 w421]
          tunnel: w406 -> [w413 w420]
          tunnel: w405 -> [_ w418]
          frame "DOWN", "LEFT", "RIGHT", "UP" {
            n159 = call "Enqueue Message.vi"("error in (no error)"=w414, "Message Data"=w412, "Message"="Key", "Message Queue"=w413) -> ("error out"=w415:errorcluster)  [unwired: 6 in, 1 out]
          }
          frame "0", Default {
            n160 = Not Equal?(x=w418, y=w417) -> (x != y?=w419:bool)
            n161 = case shown="True" w419 {
              tunnel: [w423 w427] -> w422
              tunnel: w421 -> [w423 w426]
              tunnel: w420 -> [_ w425]
              tunnel: w417 -> [_ w424]
              frame False {
              }
              frame True {
                # "bola uvolnena klavesa"
                n162 = call "Enqueue Message.vi"("error in (no error)"=w426, "Message Data"=w424, "Message"="Key", "Message Queue"=w425) -> ("error out"=w427:errorcluster)  [unwired: 6 in, 1 out]
              }
            }
          }
        }
      }
      event User Event {
        n163 = event-data() -> ()  [unwired: 1 in, 1 out]
      }
      event "Auto diode": Value Change {
        n164 = event-data() -> ("NewVal"=w431:bool)  [unwired: 1 in]
        n165 = shared-variable ".\\Inter Loop Variables.lvlib\\Auto diode"(w431) -> ()  [unwired: 1 in, 1 out]
        n166 = call "Enqueue Message.vi"("Message"="Loopback+ADA", "Message Queue"=w430) -> ("error out"=w432:errorcluster)  [unwired: 8 in, 1 out]
      }
      event "Loopback": Value Change {
        n167 = event-data() -> ("NewVal"=w435:bool)  [unwired: 1 in]
        n168 = shared-variable ".\\Inter Loop Variables.lvlib\\Loopback"(w435) -> ()  [unwired: 1 in, 1 out]
        n169 = call "Enqueue Message.vi"("Message"="Loopback+ADA", "Message Queue"=w434) -> ("error out"=w436:errorcluster)  [unwired: 8 in, 1 out]
      }
      event "LEFT", "DOWN", "RIGHT", "UP": Value Change {
        n170 = event-data() -> ()  [unwired: 1 in, 1 out]
        n171 = Build Array("RIGHT", "UP", "LEFT", "DOWN") -> (w438:bool[])
        n172 = call "Enqueue Message.vi"("Message Data"=w438, "Message"="Move", "Message Queue"=w443) -> ("error out"=w444:errorcluster)  [unwired: 7 in, 1 out]
      }
      event "Total stop": Value Change {
        w448 = TRUE  # Priority Message
        # "The UI Message Loop handles sending the Exit message to other loops."
        n173 = event-data() -> ()  [unwired: 1 in, 6 out]
        n174 = call "Enqueue Message.vi"("Priority Message? (F)"=w448, "Message"="Exit", "Message Queue"=w446) -> ("error out"=w447:errorcluster)  [unwired: 7 in, 1 out]
      }
      event Application Instance Close? {
        w453 = TRUE  # Priority Message
        n175 = event-data() -> ()  [unwired: 1 in, 5 out]
        n176 = call "Enqueue Message.vi"("Priority Message? (F)"=w453, "Message"="Exit", "Message Queue"=w451) -> ("error out"=w452:errorcluster)  [unwired: 7 in, 1 out]
        n177 = event-data("Discard?"=TRUE) -> ()  [unwired: 1 in, 1 out]
      }
      event Panel Close? {
        w458 = TRUE  # Priority Message
        n178 = event-data() -> ()  [unwired: 1 in, 4 out]
        n179 = call "Enqueue Message.vi"("Priority Message? (F)"=w458, "Message"="Exit", "Message Queue"=w456) -> ("error out"=w457:errorcluster)  [unwired: 7 in, 1 out]
        n180 = event-data("Discard?"=TRUE) -> ()  [unwired: 1 in, 1 out]
      }
    }
    n181 = case shown="Error" w389 {
      tunnel: [w399 TRUE ("Discard?")] -> w396
      tunnel: w395 -> [w399 _]
      tunnel: w393 -> [_ w400]
      frame No Error {
      }
      frame Error {
        # "On error, send Exit message, and stop loop."
        n182 = call "Enqueue Message.vi"("Priority Message? (F)"=TRUE ("Discard?"), "Message"="Exit", "Message Queue"=w400) -> ()  [unwired: 7 in, 2 out]
      }
    }
  }
  n183 = while {
    tunnel: w42 -> [w502]
    tunnel: w40 -> [w463]
    tunnel: w13 -> [w461]
    tunnel: [w460] -> w15
    stop <- w462 stop-if-true
    # "Science Logs"
    # "Display and Logging Loop"
    n184 = Dequeue Element(queue=w502) -> (element=w474:T4, error out=w465:errorcluster)  [unwired: 2 in, 2 out]
    n185 = Unbundle By Name(w474) -> ("Vertical sum"=w475:dbl, "Horizontal sum"=w472:dbl, "ADC Values"=w473:dbl[])
    n186 = call "Final Circle Drawing.vi"("picture"=w463, "Actual values"=w473, "Horizontal summary"=w472, "Vertical summary"=w475) -> ("ADC0"=→"D-     Upper diode":dbl, "ADC2"=→"A-    Left diode":dbl, "ADC1"=→"D+    Bottom diode":dbl, "ADC3"=→"A+    Right diode":dbl, "ADC Chart"=→"ADC Chart":cluster{dbl, dbl, dbl, dbl}, "Img result"=→"Output picture":picture)  [unwired: 2 in]
    n187 = Bundle("Vertical sum"=w475, "Horizontal sum"=w472) -> (→"Difference Chart":T10)  [unwired: 1 in]
    n188 = Unbundle By Name(w474) -> ("ADC Values"=w488:dbl[], "[V]"=w487:dbl, "Clouds ctrl"=w486:bool, "Cloud Det"=w484:bool, "Cloud Sens"=w482:i8, "auto Loopback"=w481:bool, "Motor Cmd"=w479:i32, "Out Cmd"=w478:i32, "Loops"=w477:u8)
    n189 = shared-variable ".\\Inter Loop Variables.lvlib\\All loop stop"() -> (w462:bool)  [unwired: 1 in, 1 out]
    n190 = call "Pointer producer consumer TimeStampGenerator.vi"() -> ("TIME Numeric"=w489:ext)  [unwired: 8 in, 2 out]
    n191 = Boolean To (0,1)(Boolean=w484) -> (0, 1=w483:i16)
    n192 = Boolean To (0,1)(Boolean=w486) -> (0, 1=w485:i16)
    n193 = Boolean To (0,1)(Boolean=w481) -> (0, 1=w480:i16)
    n194 = Build Array (concatenate)(w489, w488, w487, w485, w483, w482, w480) -> (w500:ext[])
    n195 = call "Pointer producer consumer Motor Code n Graph.vi"("DecimalMotorCode"=w479) -> ("Motor"=→"Motor Chart":cluster{dbl, i16}, "MotorSubarray"=w499:i16[])  [unwired: 6 in, 2 out]
    n196 = Insert Into Array(array=w500, new element #1=w499, new element #2=w478, new element #3=w477) -> (w476:ext[])  [unwired: 1 in]
    n197 = call "Pointer producer consumer Sound.vi"("Sound"="Sound", "Numeric"=w479) -> ()  [unwired: 9 in]
    n198 = shared-variable ".\\Inter Loop Variables.lvlib\\Data logging"() -> (w464:bool)  [unwired: 1 in, 1 out]
    n199 = Reshape Array(w476, 16 ("dimension size"), 1 ("dimension size")) -> (w493:ext[][])
    n200 = Or(x=w464, y="Data Logging\n     ON/OFF") -> (x .or. y?=w491:bool)
    n201 = call "TDMS logging.vi"("error in (no error)"=w465, "Data"=w493, "Default TDMS path"="Default TDMS path", "logg ON/OFF"=w491) -> ("error out"=w460:errorcluster, "Logg path"=→"TDMS file name/location":path)  [unwired: 6 in]
    n202 = call "Error Handler - Displey and Log Loop.vi"("error in (no error)"=w460, "Message Queue"=w461) -> ()  [unwired: 9 in, 1 out]
  }
  n203 = call "Netw loop.vi"("error in (no error)"=w8, "Queue in"=w13) -> ("error out"=w7:errorcluster)  [unwired: 9 in]
  n204 = flat-sequence {
    tunnel: w7 -> [_]
    tunnel: [w503] -> w6
    frame #0 {
      # "signal pre SCMP ze pLV je off"
      n205 = shared-variable "My Computer\\Netw Shared Variables.lvlib\\pLV"(FALSE ("pLV")) -> (error out=w503:errorcluster)  [unwired: 1 in]
    }
  }
  n206 = call-poly <vilib>:"Close Input Device.vi"("error in (no error)"=w17, "device ID"=w19) -> ("error out"=w22:errorcluster)  [unwired: 8 out]
  n207 = Unregister For Events(event registration refnum=w27, error in=w22) -> (error out=w26:errorcluster)
  n208 = Merge Errors(w26, w31) -> (w30:errorcluster)
  n209 = call "Destroy User Event - Stop.vi"("error in (no error)"=w30, "User Event - Stop"=w24) -> ("error out"=w14:errorcluster)  [unwired: 9 in]
  n210 = disable-structure shown="Disabled" {
    frame Disabled {
      n211 = case shown="True" "Help" {
        frame False {
        }
        frame True {
          n212 = call "Pointer producer consumer help.vi"() -> ()  [unwired: 12 in]
        }
      }
    }
    frame Enabled {
    }
  }
  n213 = flat-sequence {
    tunnel: [w506] -> w16
    tunnel: w15 -> [_]
    frame #0 {
      # "ukoncenie logovania v pripade ze bol \nstop a logovanie ON"
      n214 = call "TDMS logging.vi"("logg ON/OFF"=FALSE) -> ("error out"=w506:errorcluster, "Logg path"=w507:path)  [unwired: 9 in]
      n215 = local write "TDMS file name/location"(w507) -> ()
    }
  }
  n216 = Release Queue(queue=w41, error in (no error)=w37) -> (error out=w23:errorcluster)  [unwired: 1 in, 2 out]
  n217 = Merge Errors(w14, w23, w16, w6) -> (w34:errorcluster)
  n218 = call <vilib>:"Simple Error Handler.vi"("error in (no error)"=w34) -> ()  [unwired: 4 in, 5 out]
  "Version" <- "5.3.0" ("Version")
